vi "EnQcmd.vi"(6 "timeout in ms (-1)":i32, 7 "priority?":bool, 8 "error in (no error)":errorcluster, 10 "command":T1, 11 "EnQin":T2) -> (0 "error out":errorcluster, 3 "EnQout":T2, 4 "timed out?":bool)   [LabVIEW 2021]
uses:
  EnQref.ctl
  EnQcmd.ctl
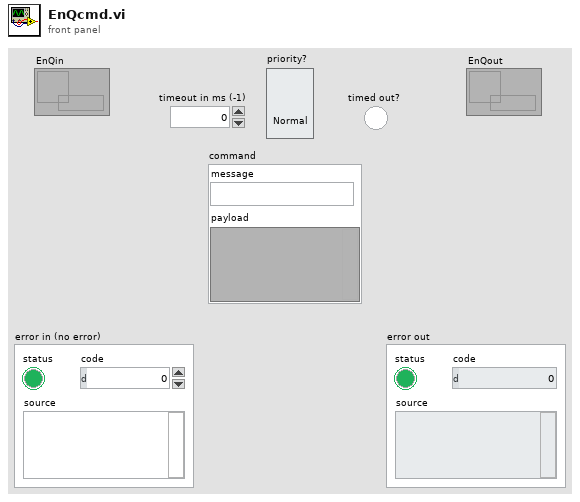
[diagram p1: front panel]
types:
  T1 = typedef "EnQcmd.ctl" = cluster{"message":string, "payload":variant}
  T2 = typedef "EnQref.ctl" = refnum<queue>
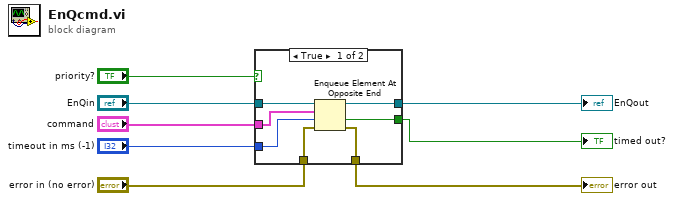
[diagram p0: block diagram]
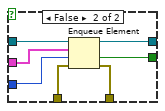
[diagram p2: hidden frame]
diagram:
  n1 = case shown="True" "priority?" {
    tunnel: "EnQin" -> [w15 w22]
    tunnel: [w14 w21] -> w8
    tunnel: "error in (no error)" -> [w13 w20]
    tunnel: [w12 w19] -> w6
    tunnel: [w11 w18] -> w5
    tunnel: "timeout in ms (-1)" -> [w10 w17]
    tunnel: "command" -> [w9 w16]
    frame True {
      n2 = Enqueue Element At Opposite End(queue=w15, element=w9, timeout in ms (-1)=w10, error in (no error)=w13) -> (queue out=w14:T2, timed out?=w11:bool, error out=w12:errorcluster)
    }
    frame False {
      n3 = Enqueue Element(queue=w22, element=w16, timeout in ms (-1)=w17, error in (no error)=w20) -> (queue out=w21:T2, timed out?=w18:bool, error out=w19:errorcluster)
    }
  }
  "error out" <- w6
  "timed out?" <- w5
  "EnQout" <- w8
